vi "PCO_SetFastTimingMode.vi"(8 "error in (no error)":errorcluster {"code" format="%x"}, 10 "wFastTimingMode":u16(ring) items=["OFF", "ON"], 11 "ph":u64) -> (0 "error out":errorcluster {"code" format="%x"}, 2 "ErrorMessage":i32 format="%x", 3 "ph out":u64)   [LabVIEW 2019, in "SDK.lvlib" / "TimingControl.lvlib"]
doc: "<b>Description:</b>\nThis function does set the fast timing mode of the camera.\n\nIf the camera is set to fast timing mode image timing is changed. The interframing time between two images is reduced to to 3.5 ìs despite the normal value of about 75 ìs. While running in fast timing mode image quality is reduced, which might be acceptable for special applications like PIV.\n\n<b>Supported camera type:</b>\npco.dimax\n\n<b>Descriptor dependency:</b>\ndwGeneralCapsDESC1: FAST_TIMING"
uses:
  TimingControl.lvlib
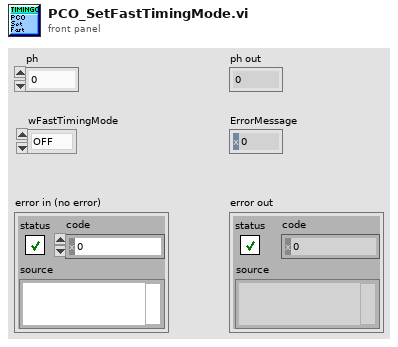
[diagram p1: front panel]
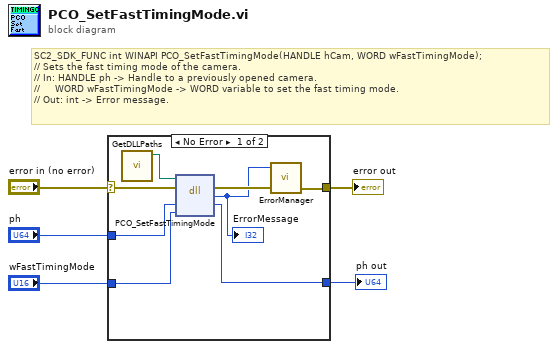
[diagram p0: block diagram]
diagram:
  # "SC2_SDK_FUNC int WINAPI PCO_SetFastTimingMode(HANDLE hCam, WORD wFastTimingMode);\n// Sets the fast timing mode of the camera.\n// In: HANDLE ph -> Handle to a previously opened camera.\n//     WORD wFastTimingMode -> WORD variable to set the fast timing mode.\n// Out: int -> Error message."
  n1 = case shown="No Error" "error in (no error)" {
    selector: "error in (no error)" -> [w10 w15]
    tunnel: "ph" -> [w13 w14]
    tunnel: [w12 w14] -> w4
    tunnel: "wFastTimingMode" -> [w11 _]
    tunnel: [w8 w15] -> w2
    frame No Error {
      n2 = call "GetDLLPaths.vi"() -> ("SC2_Cam_Path"=w6:path)  [unwired: 9 in, 2 out]
      n3 = dll-call lib="?" fn="PCO_SetFastTimingMode"(path in=w6, error in=w10, "ph"=w13, "wFastTimingMode"=w11) -> (error out=w9:errorcluster, "return type"=w7:i32, "ph"=w12:u64)  [unwired: 2 in, 1 out]
      "ErrorMessage" <- w7
      n4 = call "ErrorManager.vi"("error in (no error)"=w9, "error code"=w7) -> ("error out"=w8:errorcluster)  [unwired: 3 in]
    }
    frame Error {
    }
  }
  "ph out" <- w4
  "error out" <- w2
